vi "Configure Arming (Digits).vi"(0 "VISA resource name":refnum<visa-resource-name>, 1 "Measurement (0:Frequency)":i32(ring) items=["Frequency", "Frequency Ratio", "Period", "Totalize", "Phase", "Edge Rise Time", "Edge Fall Time", "Positive Pulse Width", "Negative Pulse Width", "Duty Cycle", "Time Interval", "Volt Maximum", "Volt Minimum"], 5 "Digits (3)":i32=3, 11 "error in (no error)":errorcluster) -> (4 "VISA resource name out":refnum<visa-resource-name>, 15 "error out":errorcluster)   [LabVIEW 2020, in "Counter.lvlib" / "PICOTEST U62XXA series.lvlib"]
doc: "Configures the parameters required for Digits Arming. Digits arming sets the number of significant digits of measurements. This VI should be called after the Configure Measurement VI.\n\n<B>Note:</B>\n\n<B>Only</B> Frequency, Frequency Ratio and Period Measurements have Digits Arming capabilities."
uses:
  PICOTEST U62XXA series.lvlib
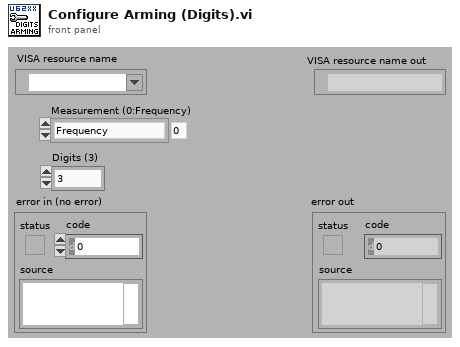
[diagram p1: front panel]
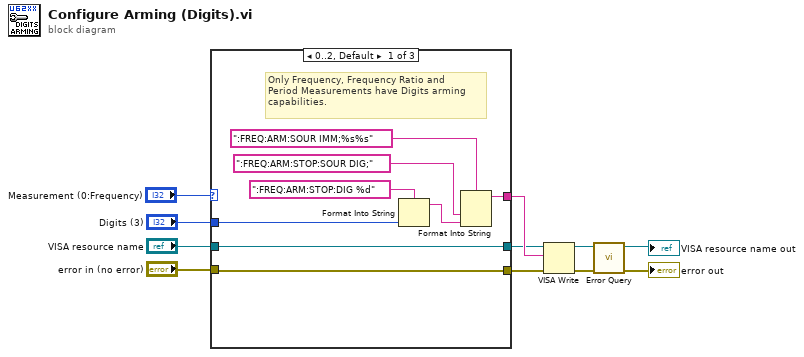
[diagram p0: block diagram]
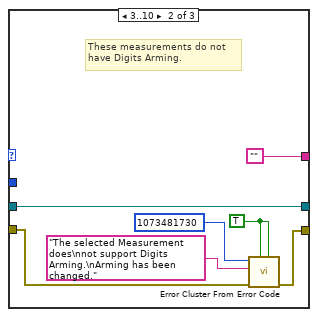
[diagram p2: hidden frame]
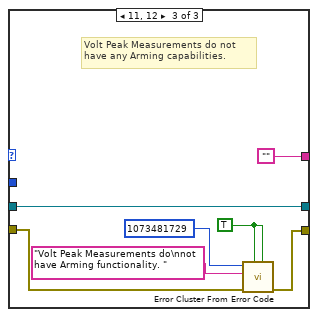
[diagram p3: hidden frame]
diagram:
  n1 = case shown="0..2, Default" "Measurement (0:Frequency)" {
    tunnel: "VISA resource name" -> [w16 w21 w28]
    tunnel: "error in (no error)" -> [w18 w23 w30]
    tunnel: [w18 w20 w27] -> w5
    tunnel: "Digits (3)" -> [w17 _ _]
    tunnel: [w15 "" ""] -> w3
    tunnel: [w16 w21 w28] -> w1
    frame 0..2, Default {
      # "Only Frequency, Frequency Ratio and\nPeriod Measurements have Digits arming\ncapabilities."
      n2 = Format Into String(format string=":FREQ:ARM:STOP:DIG %d", w17) -> (resulting string=w12:string)  [unwired: 2 in, 1 out]
      n3 = Format Into String(format string=":FREQ:ARM:SOUR IMM;%s%s", ":FREQ:ARM:STOP:SOUR DIG;" ("format string"), w12) -> (resulting string=w15:string)  [unwired: 2 in, 1 out]
    }
    frame 3..10 {
      w24 = TRUE ("is warning? (False)")
      # "These measurements do not \nhave Digits Arming."
      n4 = call <vilib>:"Error Cluster From Error Code.vi"("is warning? (False)"=w24, "show call chain? (False)"=w24, "error in (no error)"=w23, "error message (\"\")"="The selected Measurement does\nnot support Digits Arming.\nArming has been changed." ("error message (\"\")"), "error code (0)"=1073481730 ("Code")) -> ("error out"=w20:errorcluster)  [unwired: 4 in]
    }
    frame 11, 12 {
      w31 = TRUE ("is warning? (False)")
      # "Volt Peak Measurements do not \nhave any Arming capabilities."
      n5 = call <vilib>:"Error Cluster From Error Code.vi"("is warning? (False)"=w31, "show call chain? (False)"=w31, "error in (no error)"=w30, "error message (\"\")"="Volt Peak Measurements do\nnot have Arming functionality. " ("error message (\"\")"), "error code (0)"=1073481729 ("Code")) -> ("error out"=w27:errorcluster)  [unwired: 4 in]
    }
  }
  n6 = VISA Write(VISA resource name=w1, write buffer=w3, error in (no error)=w5) -> (VISA resource name out=w11:refnum<visa-resource-name>, error out=w10:errorcluster)  [unwired: 1 out]
  n7 = call "Error Query.vi"("error in (no error)"=w10, "VISA resource name"=w11) -> ("error out"=→"error out":errorcluster, "VISA resource name out"=→"VISA resource name out":refnum<visa-resource-name>)  [unwired: 6 in, 2 out]
